vi "HEWH ANSI Rate Display.vi"(4 "Raw Timer 15":dbl format="%<%H:%M:%S>t", 5 "Raw Timer 25":dbl format="%<%H:%M:%S>t", 6 "15 Min Display":string, 7 "Raw Timer 20":dbl format="%<%H:%M:%S>t", 8 "Error In":errorcluster, 9 "ANSI Rate Out":T1, 10 "20 Min Display":string, 11 "25 Min Display":string) -> (0 "Error Out":errorcluster, 2 "Raw Timer Output":dbl format="%<%H:%M:%S>t", 3 "Output Display":string)   [LabVIEW 2020]
uses:
  HEWH ANSI Rate.ctl
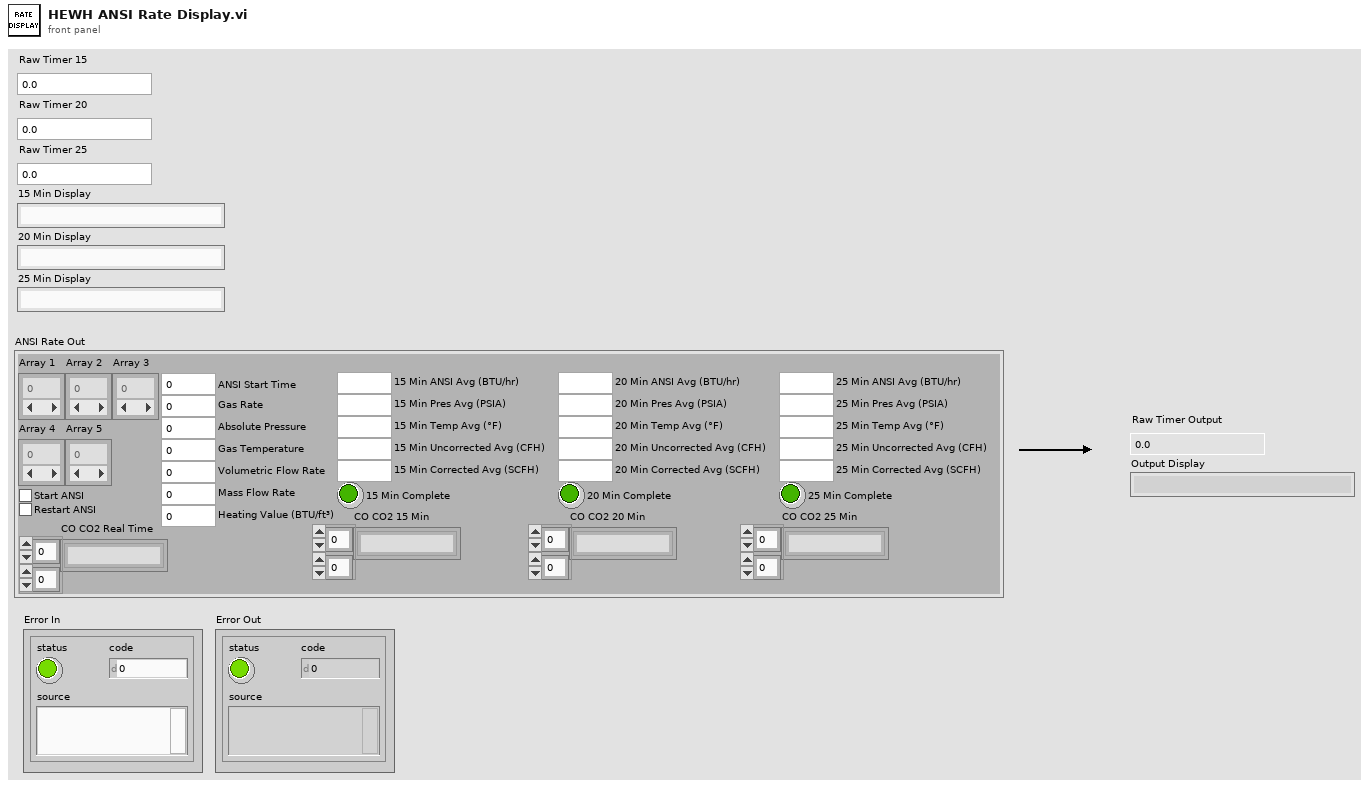
[diagram p1: front panel]
types:
  T1 = typedef "HEWH ANSI Rate.ctl" = cluster{"Array 1":dbl[], "Array 3":dbl[], "Array 2":dbl[], "Start ANSI":bool, "ANSI Start Time":dbl, "Restart ANSI":bool, "15 Min ANSI Avg (BTU/hr)":dbl, "20 Min ANSI Avg (BTU/hr)":dbl, "25 Min ANSI Avg (BTU/hr)":dbl, "Absolute Pressure":dbl, "Gas Temperature":dbl, "Volumetric Flow Rate":dbl, "Mass Flow Rate":dbl, "Array 4":dbl[], "Array 5":dbl[], "Gas Rate":dbl, "15 Min Pres Avg (PSIA)":dbl, "20 Min Pres Avg (PSIA)":dbl, "25 Min Pres Avg (PSIA)":dbl, "15 Min Temp Avg (°F) ":dbl, "20 Min Temp Avg (°F)":dbl, "25 Min Temp Avg (°F)":dbl, "15 Min Uncorrected Avg (CFH)":dbl, "20 Min Uncorrected Avg (CFH)":dbl, "25 Min Uncorrected Avg (CFH)":dbl, "15 Min Corrected Avg (SCFH)":dbl, "20 Min Corrected Avg (SCFH)":dbl, "25 Min Corrected Avg (SCFH)":dbl, "15 Min Complete":bool, "20 Min Complete":bool, "25 Min Complete":bool, "Heating Value (BTU/ft³)":dbl, "CO CO2 15 Min":string[][], "CO CO2 20 Min":string[][], "CO CO2 25 Min":string[][], "CO CO2 Real Time":string[][]}
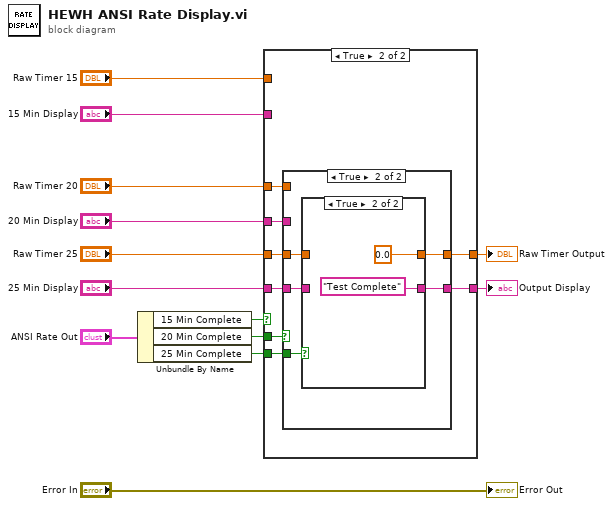
[diagram p0: block diagram]
diagram:
  n1 = Unbundle By Name("ANSI Rate Out") -> ("15 Min Complete"=w7:bool, "20 Min Complete"=w10:bool, "25 Min Complete"=w12:bool)
  n2 = case shown="True" w7 {
    tunnel: "15 Min Display" -> [w15 _]
    tunnel: [w15 w21] -> w9
    tunnel: w10 -> [_ w23]
    tunnel: "20 Min Display" -> [_ w22]
    tunnel: w12 -> [_ w20]
    tunnel: "25 Min Display" -> [_ w19]
    tunnel: "Raw Timer 15" -> [w14 _]
    tunnel: [w14 w17] -> w4
    tunnel: "Raw Timer 20" -> [_ w18]
    tunnel: "Raw Timer 25" -> [_ w16]
    frame False {
    }
    frame True {
      n3 = case shown="True" w23 {
        tunnel: w22 -> [w25 _]
        tunnel: [w25 w29] -> w21
        tunnel: w20 -> [_ w30]
        tunnel: w19 -> [_ w28]
        tunnel: w18 -> [w24 _]
        tunnel: [w24 w26] -> w17
        tunnel: w16 -> [_ w27]
        frame False {
        }
        frame True {
          n4 = case shown="True" w30 {
            tunnel: [w32 "Test Complete" ("ANSI Display")] -> w29
            tunnel: w28 -> [w32 _]
            tunnel: w27 -> [w31 _]
            tunnel: [w31 0.0] -> w26
            frame False {
            }
            frame True {
            }
          }
        }
      }
    }
  }
  "Output Display" <- w9
  "Raw Timer Output" <- w4
  "Error Out" <- "Error In"
